vi "Set Shared Regs.vi"(0 "shared in":refnum<class "niUSRP Rx Core v1 FPGA.lvclass">=refnum, 5 "shared regs":T1) -> (4 "shared out":refnum<class "niUSRP Rx Core v1 FPGA.lvclass">)   [LabVIEW 2023, in "niUSRP Rx Core v1 FPGA.lvclass"]
uses:
  <instrlib>/niUSRP/Reference FPGA/Rx Core/niUSRP Rx Core v1 FPGA.lvclass
  <instrlib>/niVST/Reference FPGA/FPGA/Shared/v1/Registers/Public/Typedefs/Shared Registers.ctl
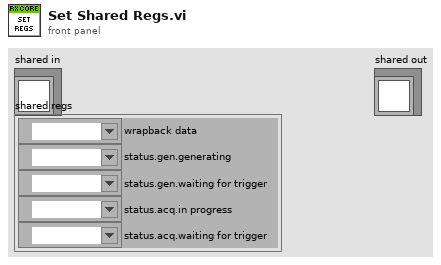
[diagram p1: front panel]
types:
  T1 = typedef "niVST Shared Registers v1 FPGA.lvclass/Shared Registers.ctl" = cluster{"wrapback data":refnum<k21>, "status.gen.generating":refnum<k21>, "status.gen.waiting for trigger":refnum<k21>, "status.acq.in progress":refnum<k21>, "status.acq.waiting for trigger":refnum<k21>}
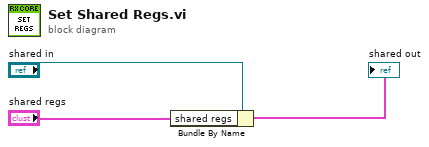
[diagram p0: block diagram]
diagram:
  n1 = Bundle By Name(cluster="shared in", "shared regs"="shared regs") -> (→"shared out":cluster{})
